vi "Configure Channel (TC Normal).vi"(0 "VISA resource name":refnum<visa-resource-name>, 5 "Channel (0001)":string="0001", 7 "Enable Channel (True)":bool=TRUE, 9 "Range and Span":T1={"Thermocouple Type (0 : R)"=0, "Enable Span (False)"=FALSE, "Lower Span (0.0)"=0.0, "Upper Span (1760.0)"=1760.0, "Bias (0)"=0.0} {"Thermocouple Type (0 : R)" items=["R", "S", "B", "K", "K-H", "E", "J", "T", "N", "W", "L", "U", "WRe3-25", "PLATINEL", "PR20-40", "KpvsAu7Fe", "NiNiMo", "WWRe26", "N14", "XK"]; "Bias (0)" min=-99999.9 max=99999.9 format="%#.1f"; "Upper Span (1760.0)" min=-10000.0 max=10000.0 format="%#.1f"; "Lower Span (0.0)" min=-10000.0 max=10000.0 format="%#.1f"}, 11 "error in (no error)":errorcluster) -> (4 "VISA resource name out":refnum<visa-resource-name>, 6 "Channel":string, 15 "error out":errorcluster)   [LabVIEW 2020, in "Yokogawa GX Series.lvlib"]
doc: "Sets the input range as thermocouple.\n\nCommand: SRangeAI"
uses:
  <instrlib>/Yokogawa GX Series/Yokogawa GX Series.lvlib
  <instrlib>/Yokogawa GX Series/Private/TC Range.vi
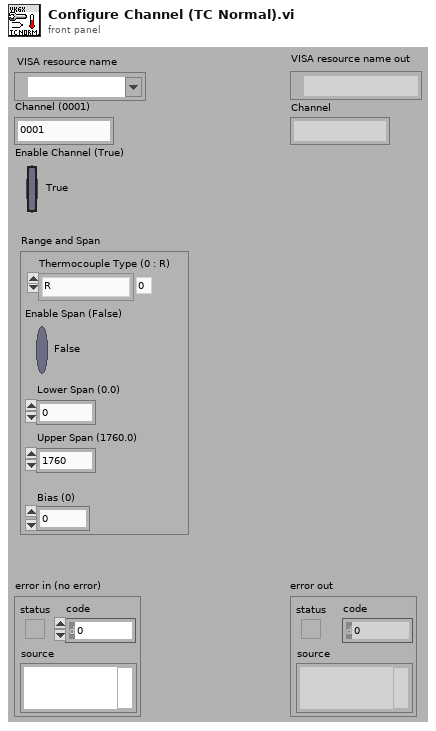
[diagram p1: front panel]
types:
  T1 = cluster{"Thermocouple Type (0 : R)":i32, "Enable Span (False)":bool, "Lower Span (0.0)":dbl, "Upper Span (1760.0)":dbl, "Bias (0)":dbl}
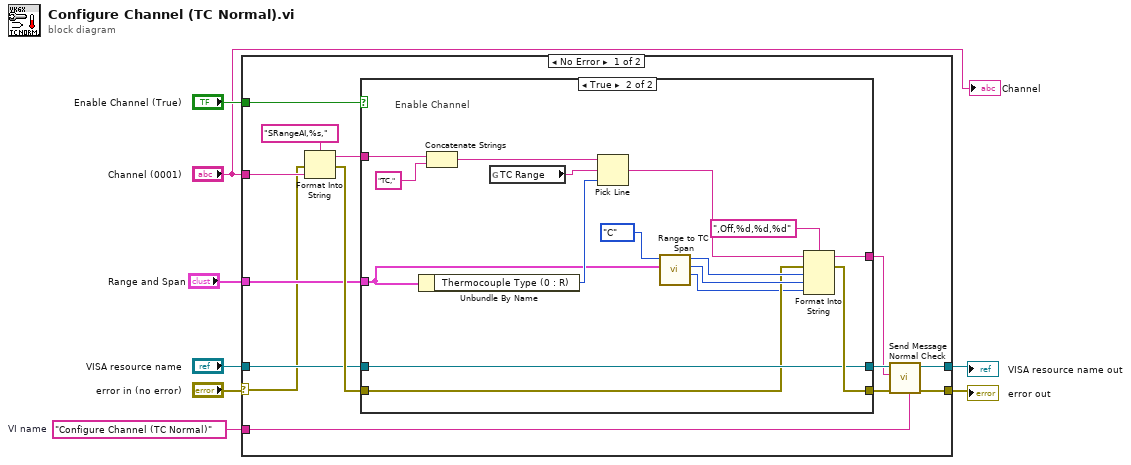
[diagram p0: block diagram]
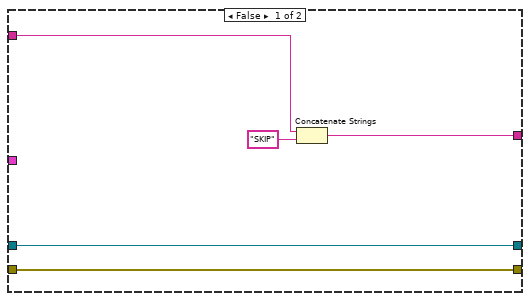
[diagram p2: hidden frame]
diagram:
  w2 = "Configure Channel (TC Normal)"  # VI name
  n1 = case shown="No Error" "error in (no error)" {
    selector: "error in (no error)" -> [w9 w44]
    tunnel: "Enable Channel (True)" -> [w19 _]
    tunnel: "VISA resource name" -> [w18 w45]
    tunnel: "Range and Span" -> [w17 _]
    tunnel: [w14 w45] -> w5
    tunnel: [w13 w44] -> w4
    tunnel: "Channel (0001)" -> [w11 _]
    tunnel: w2 -> [w10 _]
    frame No Error {
      n2 = Format Into String(format string="SRangeAI,%s,", error in=w9, w11) -> (resulting string=w20:string, error out=w21:errorcluster)  [unwired: 1 in]
      n3 = case shown="True" w19 {
        tunnel: w21 -> [w24 w33]
        tunnel: [w24 w42] -> w15
        tunnel: w20 -> [w27 w35]
        tunnel: [w26 w38] -> w12
        tunnel: w18 -> [w23 w34]
        tunnel: [w23 w34] -> w16
        tunnel: w17 -> [_ w30]
        frame False {
          n4 = Concatenate Strings(w27, "SKIP") -> (w26:string)
        }
        frame True {
          # "Enable Channel"
          n5 = Unbundle By Name(w30) -> ("Thermocouple Type (0 : R)"=w32:i32)
          n6 = Concatenate Strings(w35, "TC,") -> (w37:string)
          n7 = global read "TC Range.vi" "TC Range"() -> (w28:string)
          n8 = Pick Line(string ("")=w37, multi-line string=w28, line index=w32) -> (output string=w41:string)
          n9 = call <instrlib>:"Range to TC Span.vi"("Range and Span"=w30, "Temp. Unit (0: C)"=enum16{"C", "F"}."C") -> ("Bias"=w29:i32, "Upper Span"=w39:i32, "Lower Span"=w40:i32)  [unwired: 7 in]
          n10 = Format Into String(format string=",Off,%d,%d,%d", initial string=w41, error in=w33, w40, w39, w29) -> (resulting string=w38:string, error out=w42:errorcluster)
        }
      }
      n11 = call <instrlib>:"Send Message Normal Check.vi"("Source (\"\")"=w10, "error in (no error)"=w15, "Send Message (\"\")"=w12, "VISA resource name"=w16) -> ("error out"=w13:errorcluster, "VISA resource name out"=w14:refnum<visa-resource-name>)  [unwired: 2 in, 4 out]
    }
    frame Error {
    }
  }
  "error out" <- w4
  "VISA resource name out" <- w5
  "Channel" <- "Channel (0001)"
